vi "Serial_Number.vi"(8 "error in (no error)":errorcluster) -> (0 "error out":errorcluster, 3 "Serial Number":string)   [LabVIEW 2011]
doc: "This VI reads the serial number and converts it into proper format.\n\nInputs:\nNone\n\nOutputs:\n1.Serial Number: The serial number of the device being tested."
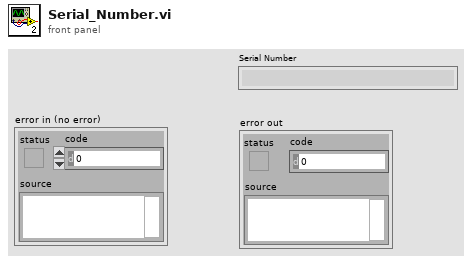
[diagram p1: front panel]
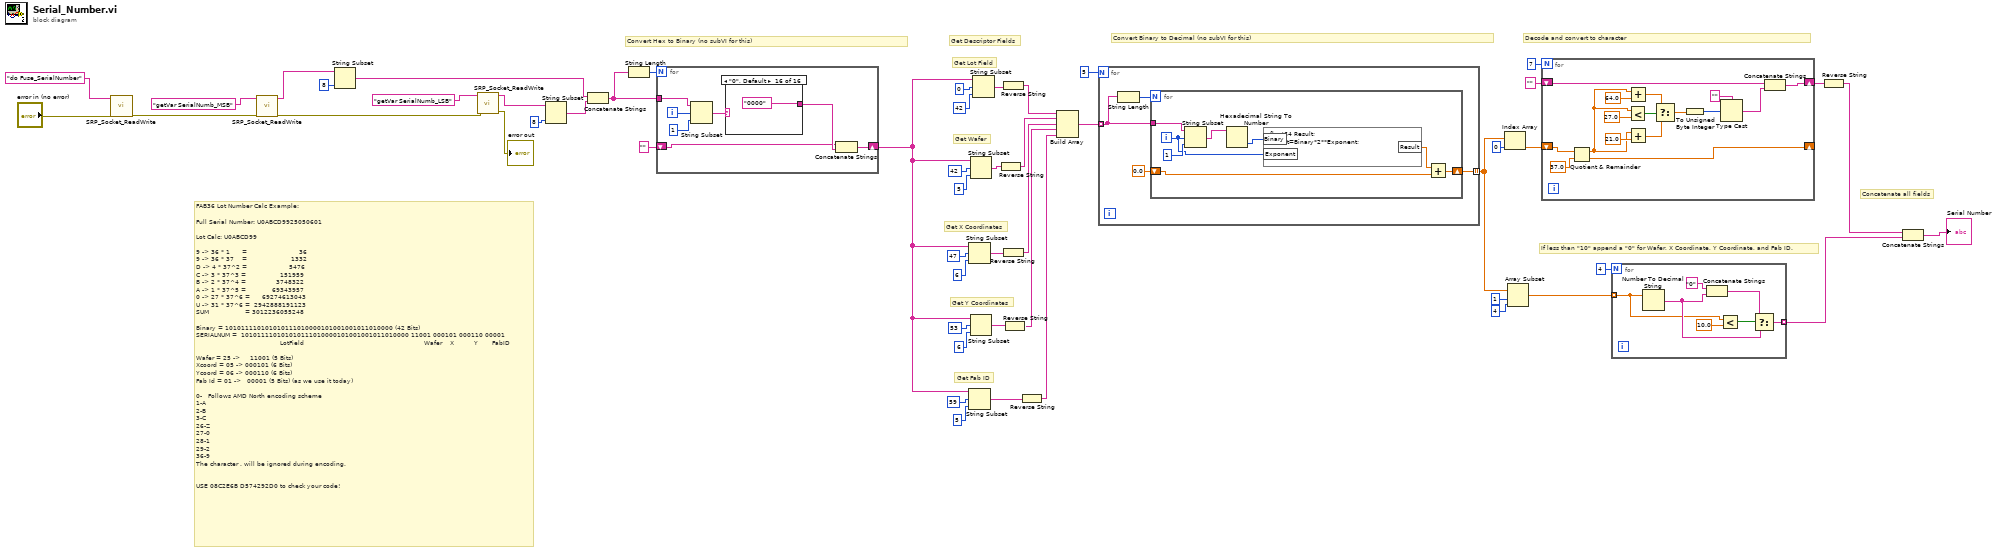
[diagram p0: block diagram]
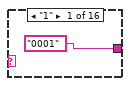
[diagram p2: hidden frame]
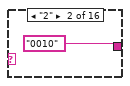
[diagram p3: hidden frame]
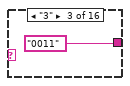
[diagram p4: hidden frame]
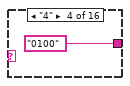
[diagram p5: hidden frame]
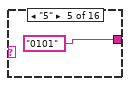
[diagram p6: hidden frame]
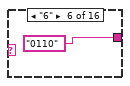
[diagram p7: hidden frame]
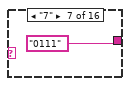
[diagram p8: hidden frame]
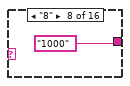
[diagram p9: hidden frame]
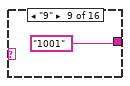
[diagram p10: hidden frame]
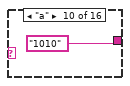
[diagram p11: hidden frame]
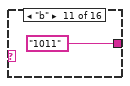
[diagram p12: hidden frame]
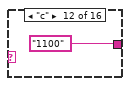
[diagram p13: hidden frame]
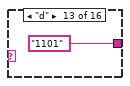
[diagram p14: hidden frame]
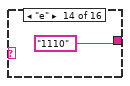
[diagram p15: hidden frame]
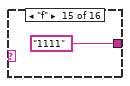
[diagram p16: hidden frame]
diagram:
  # "If less than \"10\" append a \"0\" for Wafer, X Coordinate, Y Coordinate, and Fab ID."
  # "Concatenate all fields"
  # "FAB36 Lot Number Calc Example:\n \nFull Serial Number: U0ABCD9925050601\n\nLot Calc: U0ABCD99\n\n9 -> 36 * 1      =                          36 \n9 -> 36 * 37    =                      1332\nD -> 4 * 37^2 =                     5476 \nC -> 3 * 37^3 =                 151959\nB -> 2 * 37^4 =               3748322\nA -> 1 * 37^5 =             69343957\n0 -> 27 * 37^6 =      69274613043\nU -> 31 * 37^6 =  2942888191123\nSUM                  = 3012236055248\n\nBinary = 101011110101010111010000101001001011010000 (42 Bits)\nSERIALNUM =  101011110101010111010000101001001011010000 11001 000101 000110 00001 \n                                          LotField                                                            Wafer    X          Y       FabID\n\nWafer = 25 ->     11001 (5 Bits) \nXcoord = 05 -> 000101 (6 Bits) \nYcoord = 06 -> 000110 (6 Bits) \nFab Id = 01 ->   00001 (5 Bits) (as we use it today)\n\n0-   Follows AMD North encoding scheme\n1-A\n2-B\n3-C\n26-Z\n27-0\n28-1\n29-2\n36-9\nThe character . will be ignored during encoding.\n\n\nUSE 08C2E6B D574292D0 to check your code!"
  # "Decode and convert to character"
  # "Get Descriptor Fields"
  # "Get Fab ID"
  # "Get Y Coordinates"
  # "Get X Coordinates"
  # "Get Wafer"
  # "Get Lot Field"
  # "Convert Binary to Decimal (no subVI for this)"
  # "Convert Hex to Binary (no subVI for this)"
  n1 = call "SRP_Socket_ReadWrite.vi"("error in (no error)"="error in (no error)", "Data In"="do Fuse_SerialNumber") -> ("error out"=w34:errorcluster)  [unwired: 7 in, 1 out]
  n2 = call "SRP_Socket_ReadWrite.vi"("error in (no error)"=w34, "Data In"="getVar SerialNumb_MSB") -> ("error out"=w33:errorcluster, "Data Out"=w18:string)  [unwired: 7 in]
  n3 = String Subset(string=w18, length (rest)=8 ("length (rest)")) -> (substring=w17:string)  [unwired: 1 in]
  n4 = call "SRP_Socket_ReadWrite.vi"("error in (no error)"=w33, "Data In"="getVar SerialNumb_LSB") -> ("error out"=→"error out":errorcluster, "Data Out"=w14:string)  [unwired: 7 in]
  n5 = String Subset(string=w14, length (rest)=8 ("length (rest)")) -> (substring=w13:string)  [unwired: 1 in]
  n6 = Concatenate Strings(w17, w13) -> (w49:string)
  n7 = String Length(string=w49) -> (length=w51:i32)
  n8 = for {
    N: w51 -> [_]
    tunnel: w49 -> [w58]
    shift-right: [w55] -> w12
    shift-left: "" -> [w53]
    i -> [w56]
    n9 = String Subset(string=w58, offset (0)=w56, length (rest)=1 ("length (rest)")) -> (substring=w59:string)
    n10 = case shown="\"0\", Default" w59 {
      tunnel: ["0001" "0010" "0011" "0100" "0101" "0110" "0111" "1000" "1001" "1010" "1011" "1100" "1101" "1110" "1111" "0000"] -> w54
      frame "1" {
      }
      frame "2" {
      }
      frame "3" {
      }
      frame "4" {
      }
      frame "5" {
      }
      frame "6" {
      }
      frame "7" {
      }
      frame "8" {
      }
      frame "9" {
      }
      frame "a" {
      }
      frame "b" {
      }
      frame "c" {
      }
      frame "d" {
      }
      frame "e" {
      }
      frame "f" {
      }
      frame "0", Default {
      }
    }
    n11 = Concatenate Strings(w53, w54) -> (w55:string)
  }
  n12 = String Subset(string=w12, offset (0)=47, length (rest)=6 ("length (rest)")) -> (substring=w7:string)
  n13 = String Subset(string=w12, offset (0)=59, length (rest)=5 ("length (rest)")) -> (substring=w11:string)
  n14 = String Subset(string=w12, offset (0)=42, length (rest)=5 ("length (rest)")) -> (substring=w8:string)
  n15 = String Subset(string=w12, offset (0)=53, length (rest)=6 ("length (rest)")) -> (substring=w6:string)
  n16 = String Subset(string=w12, offset (0)=0, length (rest)=42 ("length (rest)")) -> (substring=w9:string)
  n17 = Reverse String(1:w8) -> (0:w3:string)
  n18 = Reverse String(1:w9) -> (0:w2:string)
  n19 = Reverse String(1:w7) -> (0:w4:string)
  n20 = Reverse String(1:w6) -> (0:w5:string)
  n21 = Reverse String(1:w11) -> (0:w10:string)
  n22 = Build Array(w2, w3, w4, w5, w10) -> (w29:string[])
  n23 = for {
    N: 5 -> [_]
    tunnel: w29 -> [w77] mode=indexing
    tunnel: [w76] -> w24 mode=indexing
    n24 = String Length(string=w77) -> (length=w79:i32)
    n25 = for {
      N: w79 -> [_]
      tunnel: w77 -> [w87]
      shift-right: [w81] -> w76
      shift-left: 0.0 -> [w80]
      i -> [w83]
      n26 = String Subset(string=w87, offset (0)=w83, length (rest)=1 ("length (rest)")) -> (substring=w85:string)
      n27 = Hexadecimal String To Number(string=w85) -> (number=w84:u32)  [unwired: 2 in, 1 out]
      n28 = formula code="float64 Result;\nResult=Binary*2**Exponent;"("Binary"=w84, "Exponent"=w83) -> ("Result"=w82:dbl)
      n29 = Add(x=w82, y=w80) -> (x+y=w81:dbl)
    }
  }
  n30 = Index Array(array=w24, index=0) -> (element=w27:dbl)
  n31 = Array Subset(array=w24, index=1, length=4 ("index")) -> (w25:dbl[])
  n32 = for {
    N: 7 -> [_]
    shift-right: [w102] -> _
    shift-left: w27 -> [w101]
    shift-right: [w99] -> w37
    shift-left: "" -> [w98]
    n33 = Quotient & Remainder(x=w101, y=37.0) -> (x-y*floor(x/y)=w90:dbl, floor(x/y)=w102:dbl)
    n34 = Less?(x=w90, y=27.0) -> (x < y?=w95:bool)
    n35 = Add(x=w90, y=64.0) -> (x+y=w97:dbl)
    n36 = Add(x=w90, y=21.0) -> (x+y=w96:dbl)
    n37 = Select(t=w97, s=w95, f=w96) -> (s? t:f=w89:dbl)
    n38 = To Unsigned Byte Integer(number=w89) -> (unsigned 8bit integer=w88:u8)
    n39 = Type Cast(type="", x=w88) -> (*(type *) &x=w91:string)
    n40 = Concatenate Strings(w98, w91) -> (w99:string)
  }
  n41 = for {
    N: 4 -> [_]
    tunnel: [w105] -> w31 mode=indexing
    tunnel: w25 -> [w104] mode=indexing
    n42 = Number To Decimal String(number=w104) -> (decimal integer string=w106:string)  [unwired: 1 in]
    n43 = Concatenate Strings("0" ("string"), w106) -> (w107:string)
    n44 = Less?(x=w104, y=10.0) -> (x < y?=w108:bool)
    n45 = Select(t=w107, s=w108, f=w106) -> (s? t:f=w105:string)
  }
  n46 = Reverse String(1:w37) -> (0:w36:string)
  n47 = Concatenate Strings(w36, w31) -> (→"Serial Number":string)
